vi "Set_up_waveform Sine and Triang.vi"(0 "Amplitude (V)":dbl=1.0, 1 "DataSocketCluster In":T1={"Server Machine"="siskin", "Client Machine"="becard", "Data"="P2", "TimeStamp"=0.0, "Count"=0, "Target Process"="General Server"} {"TimeStamp" format="%.2f"}, 2 "0: sine, 1: triang":bool, 3 "TimeOut Time (s)":dbl=30.0 format="%.2f", 5 "Frequency (Hz)":dbl=100.0, 9 "Steps on PJVS curve":u32=100, 11 "error in (no error)":errorcluster) -> (4 "Voltage at each step on PJVS curve":dbl[](array[numeric]) format="%#_16g", 6 "Set frequency (Hz)":dbl=100.0, 10 "Returned number of steps on PJVS curve":string, 12 "Returned time interval on each step":string, 14 "Calculated time on step (smallest value is 17)":u32=100, 15 "error IO":errorcluster)   [LabVIEW 2020]
uses:
  DataSocketCluster external.ctl
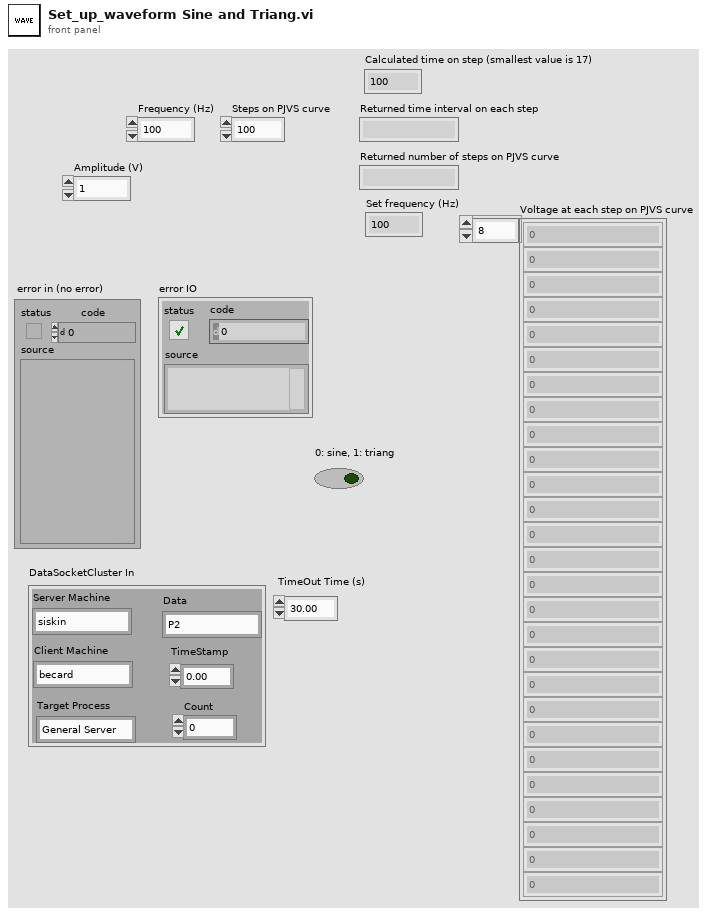
[diagram p1: front panel]
types:
  T1 = typedef "DataSocketCluster external.ctl" = cluster{"Server Machine":string, "Client Machine":string, "Data":string, "TimeStamp":dbl, "Count":i32, "Target Process":string}
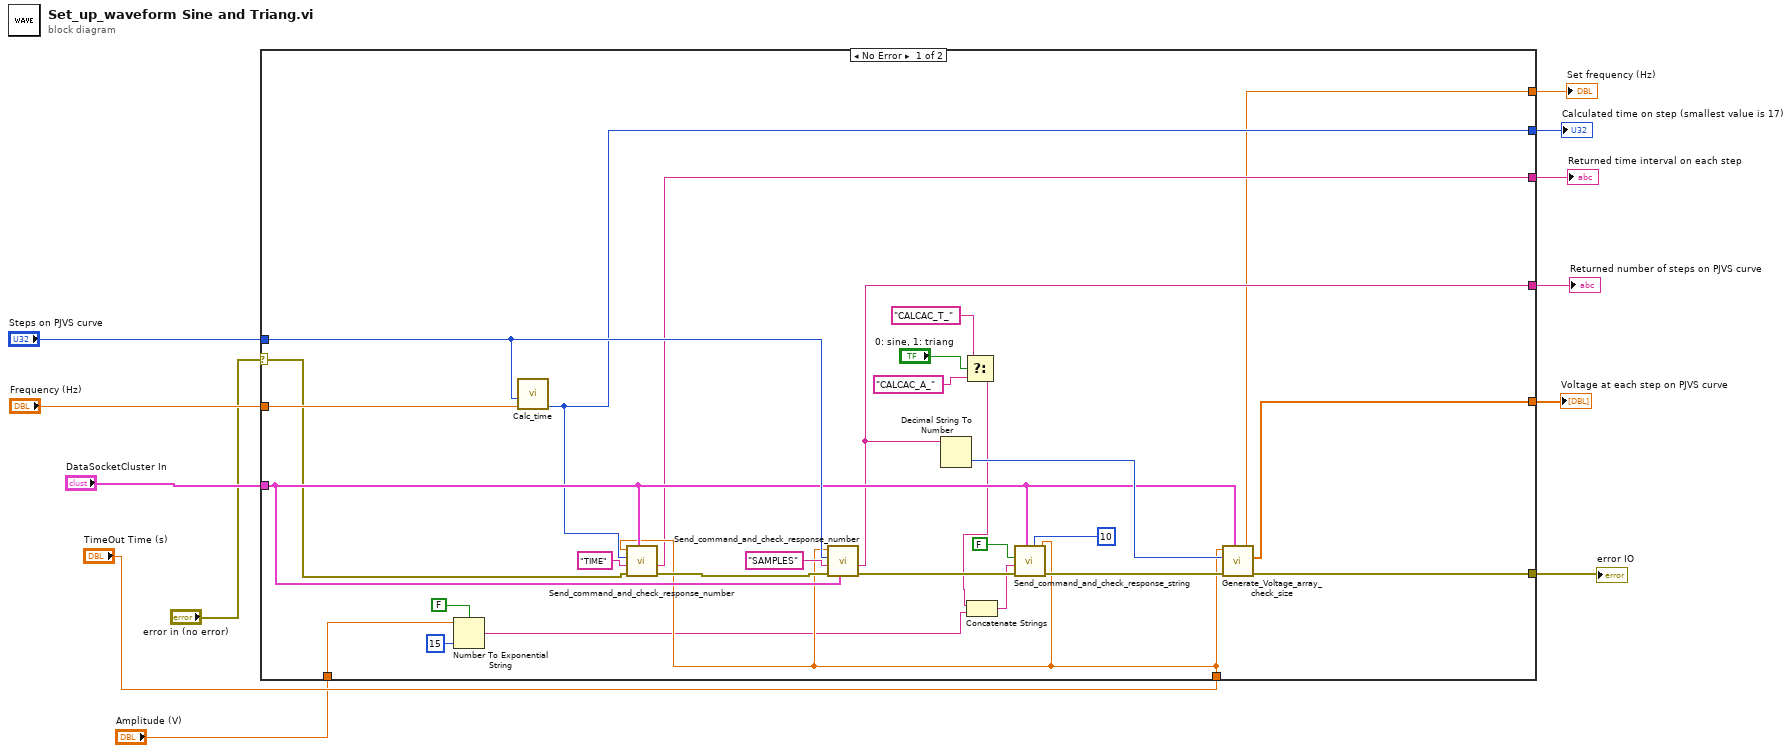
[diagram p0: block diagram]
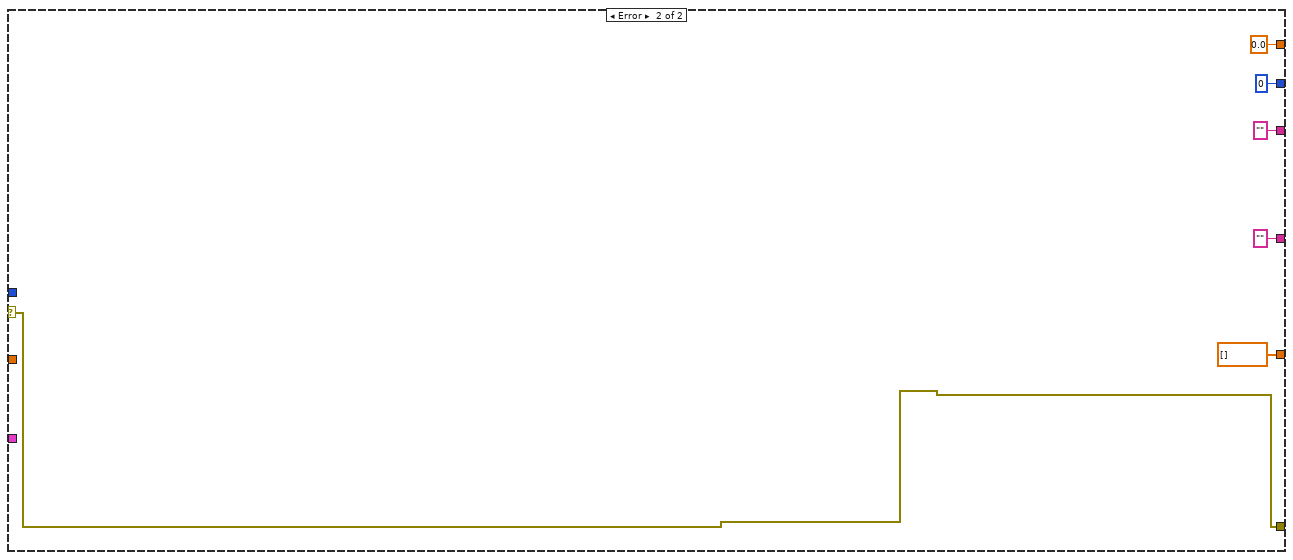
[diagram p2: hidden frame]
diagram:
  n1 = case shown="No Error" "error in (no error)" {
    selector: "error in (no error)" -> [w21 w41]
    tunnel: "Steps on PJVS curve" -> [w35 _]
    tunnel: [w30 w41] -> w12
    tunnel: "DataSocketCluster In" -> [w29 _]
    tunnel: "TimeOut Time (s)" -> [w28 _]
    tunnel: "Frequency (Hz)" -> [w27 _]
    tunnel: [w26 dbl[] [] ("Voltage at each step on PJVS curve 2")] -> w8
    tunnel: [w25 "" ("Return value")] -> w7
    tunnel: [w24 "" ("Return value")] -> w6
    tunnel: [w23 0 ("Time")] -> w5
    tunnel: [w22 0.0 ("Frequency Out (Hz)")] -> w4
    tunnel: "Amplitude (V)" -> [w18 _]
    frame No Error {
      n2 = Number To Exponential String(number=w18, precision (6)=i16 15, 1:FALSE ("use system decimal point (T)")) -> (E-format string=w17:string)  [unwired: 1 in]
      n3 = call "Calc_time.vi"("Frequency"=w27, "Steps on PJVS curve"=w35) -> ("Time"=w23:i32)  [unwired: 8 in, 1 out]
      n4 = call "Send_command_and_check_response_number.vi"("output cluster"=w29, "error in (no error)"=w21, "Command"="TIME", "Set value"=w23, "TimeOut Time (s)"=w28) -> ("error IO"=w37:errorcluster, "Return value"=w24:string)  [unwired: 3 in]
      n5 = call "Send_command_and_check_response_number.vi"("output cluster"=w29, "error in (no error)"=w37, "Command"="SAMPLES", "Set value"=w35, "TimeOut Time (s)"=w28) -> ("error IO"=w38:errorcluster, "Return value"=w25:string)  [unwired: 3 in]
      n6 = Decimal String To Number(string=w25) -> (number=w31:i32)  [unwired: 2 in, 1 out]
      n7 = Select(t="CALCAC_T_", s="0: sine, 1: triang", f="CALCAC_A_") -> (s? t:f=w13:string)
      n8 = Concatenate Strings(w13, w17) -> (w34:string)
      n9 = call "Send_command_and_check_response_string.vi"("TimeOut Time (s)"=w28, "milliseconds to wait"=u32 10, "output cluster"=w29, "error in (no error)"=w38, "Command"=w34, "test response?"=FALSE) -> ("error IO"=w39:errorcluster)  [unwired: 2 in, 1 out]
      n10 = call "Generate_Voltage_array_check_size.vi"("output cluster"=w29, "error in (no error)"=w39, "Number of Steps"=w31, "TimeOut Time (s)"=w28) -> ("error IO"=w30:errorcluster, "Voltage at each step on PJVS curve 2"=w26:dbl[], "Set Frequency"=w22:dbl)  [unwired: 1 in, 1 out]
    }
    frame Error {
    }
  }
  "error IO" <- w12
  "Voltage at each step on PJVS curve" <- w8
  "Returned number of steps on PJVS curve" <- w7
  "Returned time interval on each step" <- w6
  "Calculated time on step (smallest value is 17)" <- w5
  "Set frequency (Hz)" <- w4
